vi "BRig_Host__Loop_Consumer_RunState__closeLoop_getData_dataTS.vi"(10 "input_idx":i32[](array[numeric]), 11 "input_dataTS":u16[][](array[numeric])) -> (3 "output_dataTS":u16[][](array[numeric]))   [LabVIEW 2014]
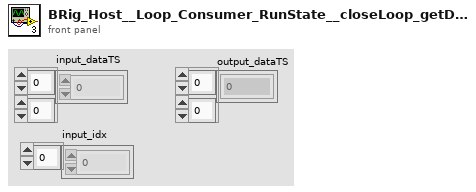
[diagram p1: front panel]
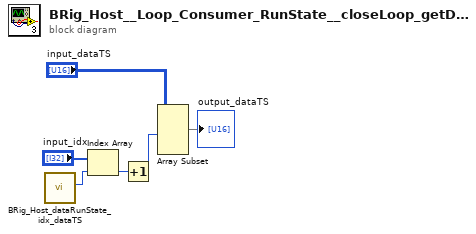
[diagram p0: block diagram]
diagram:
  n1 = call "BRig_Host_dataRunState_idx_dataTS.vi"() -> ("output_idx_dataTS"=w5:i32)  [unwired: 11 in]
  n2 = Index Array(array="input_idx", index=w5) -> (element=w2:i32)
  n3 = Increment(x=w2) -> (x+1=w4:i32)
  n4 = Array Subset(array="input_dataTS", length (row)=w4) -> (→"output_dataTS":u16[][])  [unwired: 3 in]
